vi "Fixed overlay array indexing_GD&T.vi"(11 "Overlay coordinates":cluster{"X":dbl, "Y":dbl}[](array[cluster])) -> (3 "Overlay coordinates cluster":T1)   [LabVIEW 2019]
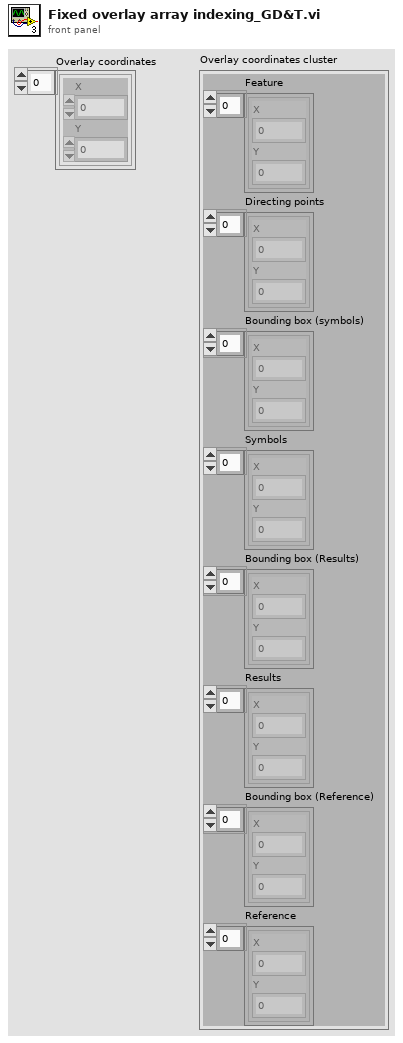
[diagram p1: front panel]
types:
  T1 = cluster{"Feature":cluster{"X":dbl, "Y":dbl}[], "Directing points":cluster{"X":dbl, "Y":dbl}[], "Bounding box (symbols)":cluster{"X":dbl, "Y":dbl}[], "Symbols":cluster{"X":dbl, "Y":dbl}[], "Bounding box (Results)":cluster{"X":dbl, "Y":dbl}[], "Results":cluster{"X":dbl, "Y":dbl}[], "Bounding box (Reference)":cluster{"X":dbl, "Y":dbl}[], "Reference":cluster{"X":dbl, "Y":dbl}[]}
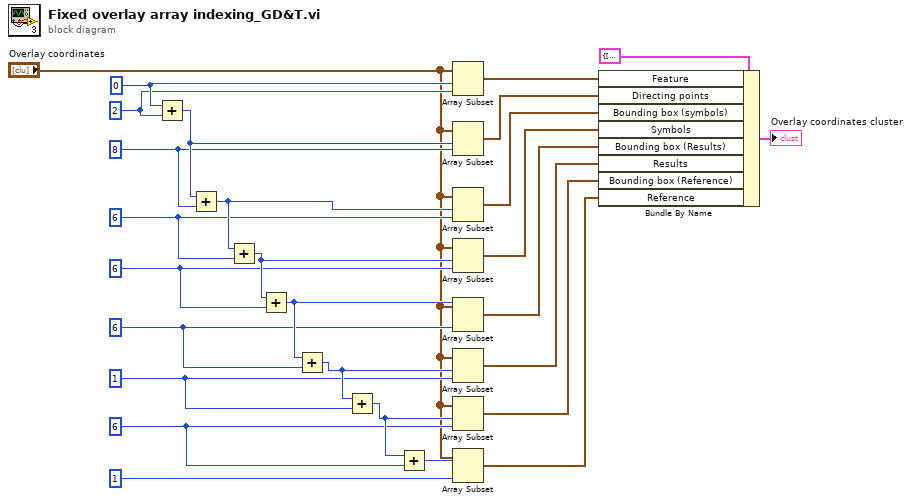
[diagram p0: block diagram]
diagram:
  w7 = 6 ("length")
  w8 = 1 ("length")
  w18 = 6 ("length")
  w20 = 6 ("length")
  w22 = 6 ("y")
  w24 = 8 ("y")
  w27 = 0 ("index")
  w26 = 2 ("length")
  n1 = Add(x=w27, y=w26) -> (x+y=w25:i32)
  n2 = Add(x=w25, y=w24) -> (x+y=w23:i32)
  n3 = Add(x=w23, y=w22) -> (x+y=w21:i32)
  n4 = Add(x=w21, y=w20) -> (x+y=w19:i32)
  n5 = Add(x=w19, y=w18) -> (x+y=w17:i32)
  n6 = Add(x=w17, y=w8) -> (x+y=w9:i32)
  n7 = Add(x=w9, y=w7) -> (x+y=w6:i32)
  n8 = Array Subset(array="Overlay coordinates", index=w27, length=w26) -> (w15:cluster{"X":dbl, "Y":dbl}[])
  n9 = Array Subset(array="Overlay coordinates", index=w25, length=w24) -> (w14:cluster{"X":dbl, "Y":dbl}[])
  n10 = Array Subset(array="Overlay coordinates", index=w23, length=w22) -> (w13:cluster{"X":dbl, "Y":dbl}[])
  n11 = Array Subset(array="Overlay coordinates", index=w21, length=w20) -> (w12:cluster{"X":dbl, "Y":dbl}[])
  n12 = Array Subset(array="Overlay coordinates", index=w19, length=w18) -> (w11:cluster{"X":dbl, "Y":dbl}[])
  n13 = Array Subset(array="Overlay coordinates", index=w17, length=w8) -> (w10:cluster{"X":dbl, "Y":dbl}[])
  n14 = Array Subset(array="Overlay coordinates", index=w9, length=w7) -> (w4:cluster{"X":dbl, "Y":dbl}[])
  n15 = Array Subset(array="Overlay coordinates", index=w6, length=1) -> (w3:cluster{"X":dbl, "Y":dbl}[])
  n16 = Bundle By Name(cluster=T1 {"Feature"=[], "Directing points"=[], "Bounding box (symbols)"=[], "Symbols"=[], "Bounding box (Results)"=[], "Results"=[], "Bounding box (Reference)"=[], "Reference"=[]} ("Overlay coordinates cluster"), "Feature"=w15, "Directing points"=w14, "Bounding box (symbols)"=w13, "Symbols"=w12, "Bounding box (Results)"=w11, "Results"=w10, "Bounding box (Reference)"=w4, "Reference"=w3) -> (→"Overlay coordinates cluster":T1)
